vi "Laboratory_practice2.vi"() -> ()   [LabVIEW 2022 SP3]
panel:
  out "Biggest":dbl
  in  "Input":dbl
  in  "Input":dbl
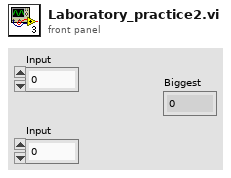
[diagram p1: front panel]
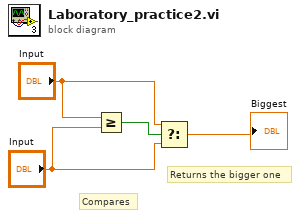
[diagram p0: block diagram]
diagram:
  # "Returns the bigger one"
  # "Compares"
  n1 = Greater Or Equal?(x="Input", y="Input") -> (x >= y?=w4:bool)
  n2 = Select(t="Input", s=w4, f="Input") -> (s? t:f=→"Biggest":dbl)
